vi "Initialise.vi"(4 "Direction":T1, 6 "Snake Colour":u32(colorbox), 8 "error in (no error)":errorcluster, 10 "Starting Elements":i32) -> (0 "error out":errorcluster, 3 "Snake out":refnum<class "Snake.lvclass">)   [LabVIEW 2018, in "Snake.lvclass"]
uses:
  Snake.lvclass
  Type Defs/Direction.ctl
  Snake.lvclass/Snake.ctl
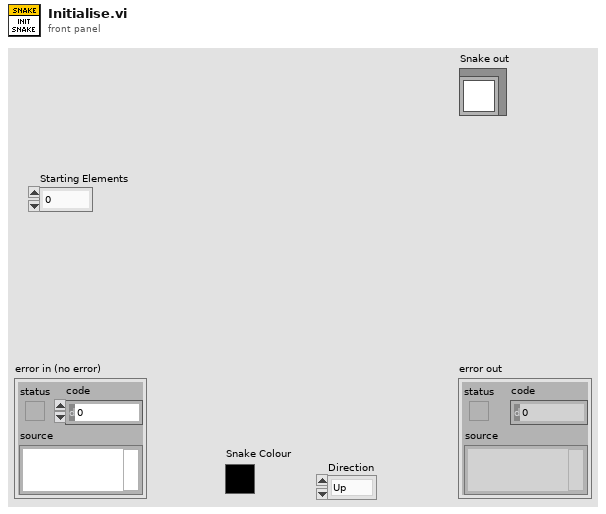
[diagram p1: front panel]
types:
  T1 = typedef "Direction.ctl" = enum16{"Up", "Down", "Left", "Right"}
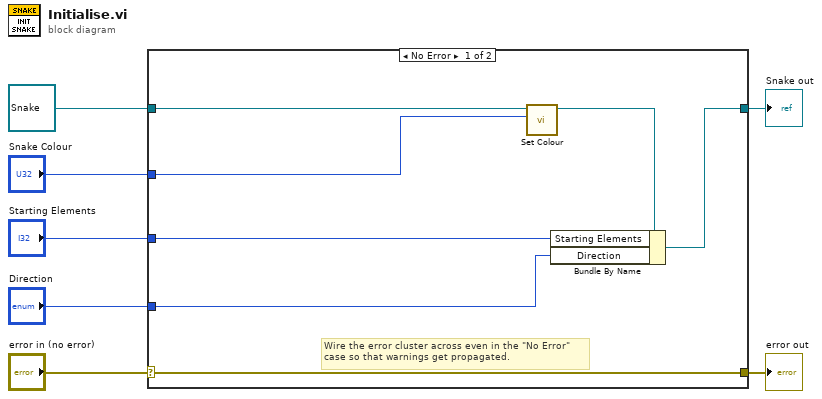
[diagram p0: block diagram]
diagram:
  n1 = case shown="No Error" "error in (no error)" {
    selector: "error in (no error)" -> [w14 w16]
    tunnel: [w14 w16] -> w6
    tunnel: [w13 w15] -> w4
    tunnel: refnum<class "Snake.lvclass"> refnum ("Snake in") -> [w11 w15]
    tunnel: "Direction" -> [w12 _]
    tunnel: "Snake Colour" -> [w9 _]
    tunnel: "Starting Elements" -> [w8 _]
    frame No Error {
      # "Wire the error cluster across even in the \"No Error\"\ncase so that warnings get propagated."
      n2 = call-dynamic "Set Colour.vi"("Componant Colour"=w9, "Game Componants in"=w11) -> ("Game Componants out"=w10:refnum<class "Snake.lvclass">)  [unwired: 9 in]
      n3 = Bundle By Name(cluster=w10, "Starting Elements"=w8, "Direction"=w12) -> (w13:refnum<class "Snake.lvclass">)
    }
    frame Error {
    }
  }
  "error out" <- w6
  "Snake out" <- w4
